vi "WSVCAP SHL FPGA LL SPI Read Data.vi"(11 "error in (no error)":errorcluster, 12 "Socket Mask":u16) -> (4 "Word Out (1-Bit for Each Channel)":u16, 15 "error out":errorcluster)   [LabVIEW 2012]
uses:
  WSVCAP SHL FPGA LL SPI Debug Global.vi
  <vilib>/eio/EIONode/EIONode.xnode
  <vilib>/rvi/eio/common/nirviEmuTemplateMethod_errors.vi
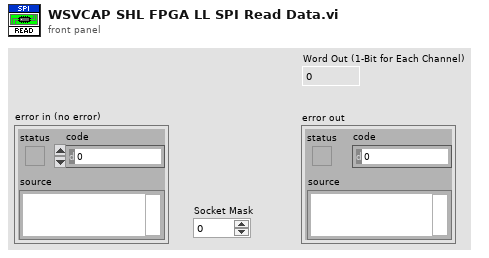
[diagram p1: front panel]
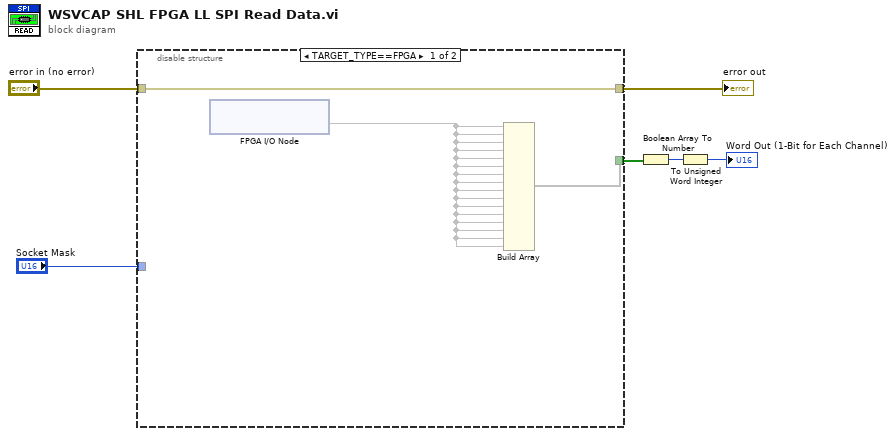
[diagram p0: block diagram]
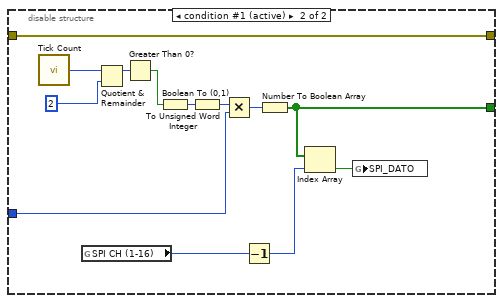
[diagram p2: hidden frame]
diagram:
  n1 = disable-structure shown="TARGET_TYPE==FPGA" {
    disable-tunnel: [w9 w11] -> w2
    disable-tunnel: [w8 w19] -> w6
    disable-tunnel: "error in (no error)" -> [w8 w19]
    disable-tunnel: "Socket Mask" -> [_ w15]
    frame condition #0 {
      n2 = xnode "FPGA I/O Node"() -> ("RFFE_DATO_S1"=w7)  [unwired: 1 in, 1 out]
      n3 = Build Array(w7, w7, w7, w7, w7, w7, w7, w7, w7, w7, w7, w7, w7, w7, w7, w7) -> (w9:void[])
    }
    frame condition #1 (active) {
      n4 = call "Tick Count"() -> ("Tick Count(Ticks)"=w22:u32)
      n5 = global read "WSVCAP SHL FPGA LL SPI Debug Global.vi" "SPI CH (1-16)"() -> (w13:i32)
      n6 = Quotient & Remainder(x=w22, y=u32 2) -> (x-y*floor(x/y)=w21:u32)  [unwired: 1 out]
      n7 = Greater Than 0?(x=w21) -> (x > 0?=w18:bool)
      n8 = Boolean To (0,1)(Boolean=w18) -> (0, 1=w17:i16)
      n9 = To Unsigned Word Integer(number=w17) -> (unsigned 16bit integer=w16:u16)
      n10 = Multiply(x=w16, y=w15) -> (x*y=w14:u16)
      n11 = Decrement(x=w13) -> (x-1=w10:i32)
      n12 = Number To Boolean Array(number=w14) -> (Boolean array=w11:bool[])
      n13 = Index Array(array=w11, index=w10) -> (element=w12:bool)
      n14 = global write "WSVCAP SHL FPGA LL SPI Debug Global.vi" "SPI_DATO"(w12) -> ()
    }
  }
  "error out" <- w6
  n15 = Boolean Array To Number(Boolean array=w2) -> (number=w3:u16)
  n16 = To Unsigned Word Integer(number=w3) -> (unsigned 16bit integer=→"Word Out (1-Bit for Each Channel)":u16)
